vi "frontEnd.vi"(8 "error in (no error)":errorcluster, 11 "WinX32Settings in":refnum<class "WinX32Settings.lvclass">) -> (0 "error out":errorcluster, 3 "WinX32Settings out":refnum<class "WinX32Settings.lvclass">)   [LabVIEW 2011, in "Tools.lvlib" / "Settings.lvlib" / "WinX32Settings.lvclass"]
uses:
  WinX32Settings.lvclass
  WinX32Settings.lvclass/WinX32Settings.ctl
  Settings.lvlib
panel:
  in  "Camera":enum16{"Pixis", "ProEM", "PixelFly"}(ring)=enum."ProEM"
  in  "Close":bool
  in  "Save Images":bool
  in  "Save as":bool
  out "Path":path
  in  "image_number":i32 caption="Image Number"
  in  "Open":bool
  in  "Save":bool
  in  "Triggering":bool
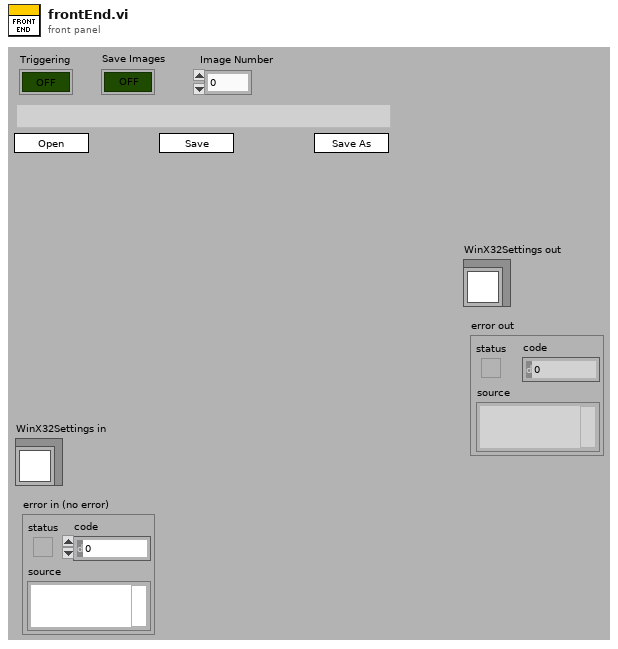
[diagram p1: front panel]
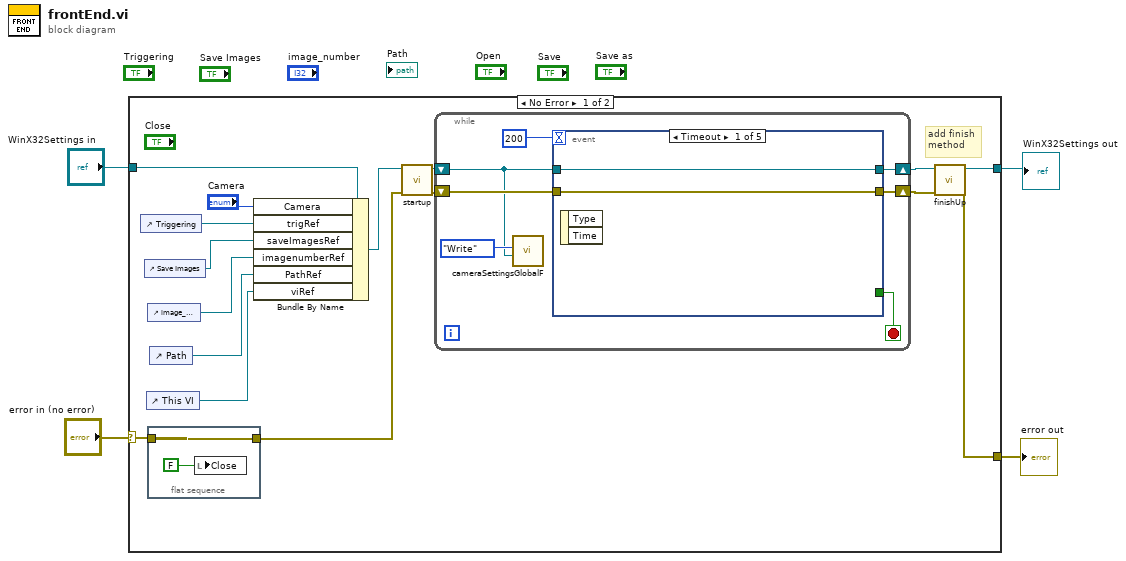
[diagram p0: block diagram]
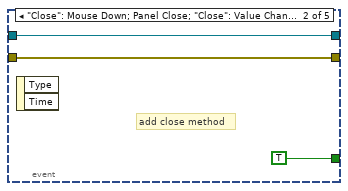
[diagram p2: hidden frame]
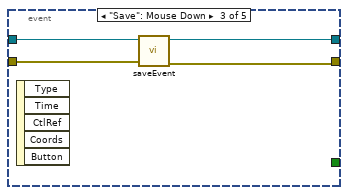
[diagram p3: hidden frame]
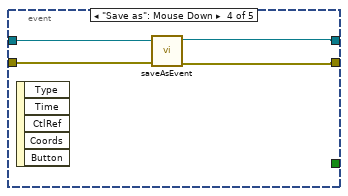
[diagram p4: hidden frame]
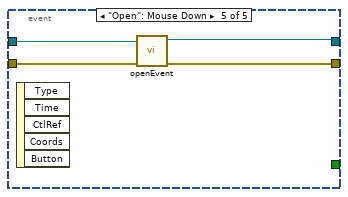
[diagram p5: hidden frame]
diagram:
  n1 = case shown="No Error" "error in (no error)" {
    selector: "error in (no error)" -> [w14 w48]
    tunnel: "WinX32Settings in" -> [w15 w47]
    tunnel: [w7 w48] -> w2
    tunnel: [w6 w47] -> w1
    frame No Error {
      # "add finish\nmethod"
      n2 = control-ref of="Triggering"() -> (w20:refnum<vi>)
      n3 = control-ref of="Save Images"() -> (w19:refnum<vi>)
      n4 = control-ref of="This VI"() -> (w16:refnum<vi>)
      n5 = control-ref of="image_number"() -> (w18:refnum<vi>)
      n6 = flat-sequence {
        tunnel: w14 -> [w21]
        tunnel: [w21] -> w11
        frame #0 {
          n7 = local write "Close"(FALSE) -> ()
        }
      }
      n8 = control-ref of="Path"() -> (w17:refnum<vi>)
      n9 = Bundle By Name(cluster=w15, "Camera"="Camera", "trigRef"=w20, "saveImagesRef"=w19, "imagenumberRef"=w18, "PathRef"=w17, "viRef"=w16) -> (w12:refnum<class "WinX32Settings.lvclass">)
      n10 = call "startup.vi"("error in (no error)"=w11, "WinX32Settings in"=w12) -> ("error out"=w10:errorcluster, "WinX32Settings out"=w13:refnum<class "WinX32Settings.lvclass">)  [unwired: 8 in]
      n11 = while {
        shift-right: [w27] -> w8
        shift-left: w10 -> [w28]
        shift-right: [w29] -> w9
        shift-left: w13 -> [w24]
        stop <- w26 stop-if-true
        n12 = call "cameraSettingsGlobalF.vi"("CamaraSettings"=w24, "Action"=enum16{"Write", "Read"}."Write") -> ()  [unwired: 9 in, 1 out]
        n13 = event shown="[0] Timeout" {
          selector: _ -> [_ _ _ _ _]
          dyn-events: _ -> [_ _ _ _ _]
          timeout: 200 -> [_ _ _ _ _]
          tunnel: [w31 w34 w36 w40 w45] -> w29
          tunnel: w24 -> [w31 w34 w38 w42 w46]
          tunnel: w28 -> [w30 w33 w37 w41 w44]
          tunnel: [w30 w33 w35 w39 w43] -> w27
          tunnel: [_ TRUE _ _ _] -> w26
          event Timeout {
            n14 = event-data() -> ()  [unwired: 1 in, 2 out]
          }
          event "Close": Mouse Down; Panel Close; "Close": Value Change {
            # "add close method"
            n15 = event-data() -> ()  [unwired: 1 in, 2 out]
          }
          event "Save": Mouse Down {
            n16 = event-data() -> ()  [unwired: 1 in, 5 out]
            n17 = call "saveEvent.vi"("error in (no error)"=w37, "WinX32Settings in"=w38) -> ("error out"=w35:errorcluster, "WinX32Settings out"=w36:refnum<class "WinX32Settings.lvclass">)  [unwired: 8 in]
          }
          event "Save as": Mouse Down {
            n18 = event-data() -> ()  [unwired: 1 in, 5 out]
            n19 = call "saveAsEvent.vi"("error in (no error)"=w41, "WinX32Settings in"=w42) -> ("error out"=w39:errorcluster, "WinX32Settings out"=w40:refnum<class "WinX32Settings.lvclass">)  [unwired: 8 in]
          }
          event "Open": Mouse Down {
            n20 = event-data() -> ()  [unwired: 1 in, 5 out]
            n21 = call "openEvent.vi"("error in (no error)"=w44, "WinX32Settings in"=w46) -> ("error out"=w43:errorcluster, "WinX32Settings out"=w45:refnum<class "WinX32Settings.lvclass">)  [unwired: 8 in]
          }
        }
      }
      n22 = call "finishUp.vi"("error in (no error)"=w8, "WinX32Settings in"=w9) -> ("error out"=w7:errorcluster, "WinX32Settings out"=w6:refnum<class "WinX32Settings.lvclass">)  [unwired: 8 in]
    }
    frame Error {
    }
  }
  "error out" <- w2
  "WinX32Settings out" <- w1
